vi "LIA Vrms2 to dBm.vi"(11 "Power Spectrum / PSD":cluster{"f0":dbl, "df":dbl, "magnitude":dbl[]}) -> (3 "Power Spectrum / PSD (dBm)":cluster{"f0":dbl, "df":dbl, "magnitude":dbl[]})   [LabVIEW 2017]
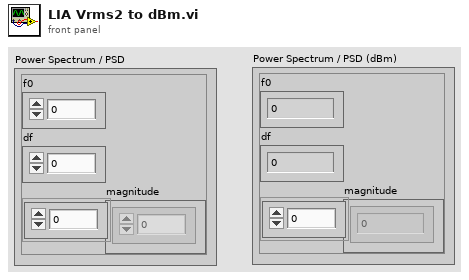
[diagram p1: front panel]
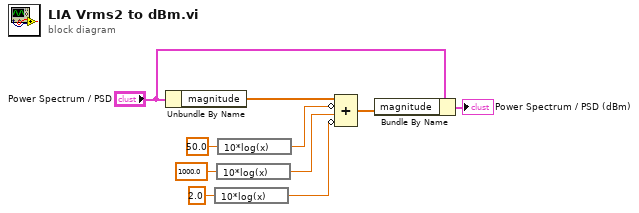
[diagram p0: block diagram]
diagram:
  n1 = Unbundle By Name("Power Spectrum / PSD") -> ("magnitude"=w7:dbl[])
  n2 = expression code="10*log(x)"(2.0) -> (w1:dbl)
  n3 = expression code="10*log(x)"(1000.0) -> (w3:dbl)
  n4 = expression code="10*log(x)"(50.0) -> (w6:dbl)
  n5 = Compound Arithmetic op=ADD(w7, invert w6, w3, invert w1) -> (w8:dbl[])
  n6 = Bundle By Name(cluster="Power Spectrum / PSD", "magnitude"=w8) -> (→"Power Spectrum / PSD (dBm)":cluster{"f0":dbl, "df":dbl, "magnitude":dbl[]})
